vi "DCA Update Limit Listbox.vi"(6 "Colors":cluster{"Pass":u32, "Fail":u32, "Nop":u32}={"Pass"=6618880, "Fail"=16711680, "Nop"=16777226}, 7 "State (Pass/Fail)":enum16{"Reset", "In Progress", "Pass/Fail"}(ring)=enum."Pass/Fail", 8 "error in (no error)":errorcluster, 9 "Pass/Fail":bool[](array[boolean]), 10 "Limits":T1[](array[typedef]), 11 "Limit Status Ref":refnum<vi>) -> (0 "error out":errorcluster, 3 "Limit Status Ref Out":refnum<vi>)   [LabVIEW 2011]
uses:
  TypeDefs/DCA Limit.ctl
  TypeDefs/DCA Limit Quantity.ctl
  TypeDefs/DCA Limit Comparison.ctl
  TypeDefs/DCA Limit Operation.ctl
  Test Referential Limit.ctl
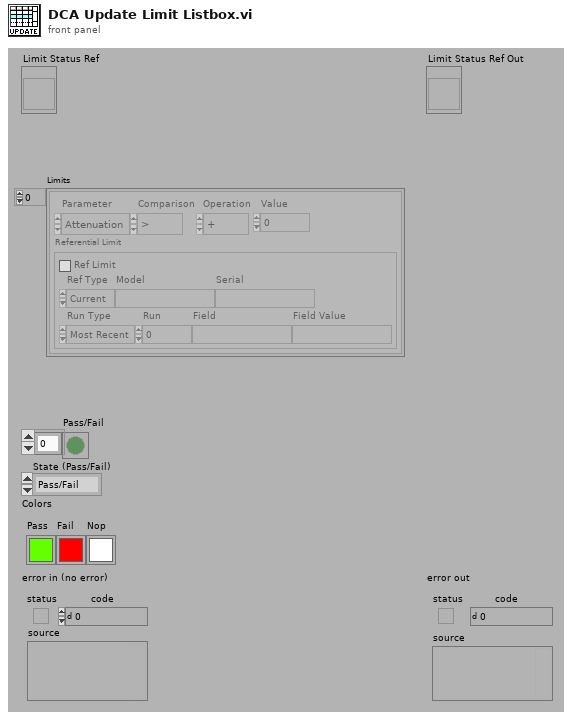
[diagram p1: front panel]
types:
  T1 = typedef "DCA Limit.ctl" = cluster{"Parameter":T2, "Comparison":T3, "Operation":T4, "Value":dbl, "Referential Limit":T5}
  T2 = typedef "DCA Limit Quantity.ctl" = enum16{"Attenuation", "Zin", "Zout", "R1", "R2", "R3", "Rab", "Rac", "Rbc"}
  T3 = typedef "DCA Limit Comparison.ctl" = enum16{">", ">=", "<", "<="}
  T4 = typedef "DCA Limit Operation.ctl" = enum16{"+", "-"}
  T5 = typedef "Test Referential Limit.ctl" = cluster{"Ref Limit":bool, "Ref Type":enum16{"Current", "Specify"}, "Model":string, "Serial":string, "Run Type":enum16{"Most Recent", "Run #", "Match Field"}, "Run":i32, "Field":string, "Field Value":string}
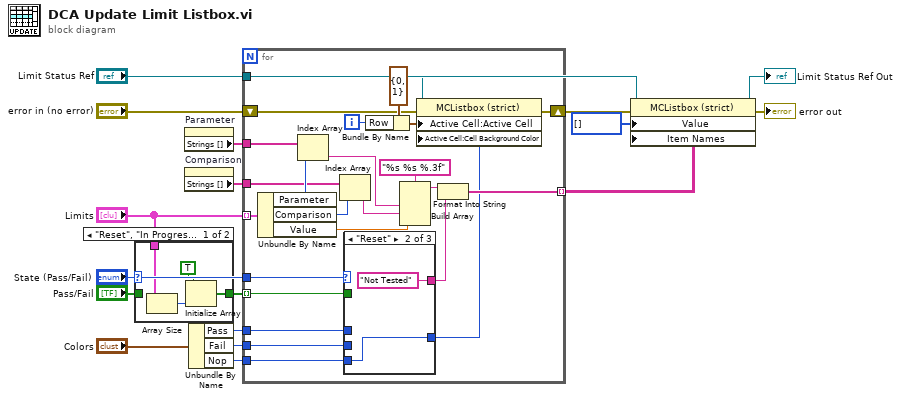
[diagram p0: block diagram]
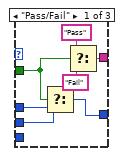
[diagram p3: hidden frame]
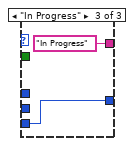
[diagram p4: hidden frame]
diagram:
  n1 = case shown="\"Reset\", \"In Progress\"" "State (Pass/Fail)" {
    tunnel: [w19 w22] -> w4
    tunnel: "Pass/Fail" -> [_ w22]
    tunnel: "Limits" -> [w18 _]
    frame "Reset", "In Progress" {
      n2 = Array Size(array=w18) -> (size(s)=w21:i32)
      n3 = Initialize Array(TRUE, w21) -> (w19:bool[])
    }
    frame "Pass/Fail" {
    }
  }
  n4 = property on="Parameter" class="Enum (strict)"() -> ("Strings []"=w9:string[])  [unwired: 2 in, 2 out]
  n5 = property on="Comparison" class="Enum (strict)"() -> ("Strings []"=w10:string[])  [unwired: 2 in, 2 out]
  n6 = Unbundle By Name("Colors") -> ("Pass"=w16:u32, "Fail"=w15:u32, "Nop"=w8:u32)
  n7 = for {
    tunnel: w16 -> [w27]
    tunnel: w15 -> [w26]
    tunnel: "Limit Status Ref" -> [w44]
    shift-right: [w42] -> w13
    shift-left: "error in (no error)" -> [w43]
    tunnel: "Limits" -> [w41] mode=indexing
    tunnel: [w39] -> w7 mode=indexing
    tunnel: w10 -> [w34]
    tunnel: w9 -> [w33]
    tunnel: w4 -> [w25] mode=indexing
    tunnel: w8 -> [w23]
    tunnel: "State (Pass/Fail)" -> [w24]
    i -> [w40]
    n8 = Unbundle By Name(w41) -> ("Parameter"=w35:T2, "Comparison"=w36:T3, "Value"=w30:dbl)
    n9 = Index Array(array=w33, index=w35) -> (element=w31:string)
    n10 = Index Array(array=w34, index=w36) -> (element=w32:string)
    n11 = case shown="\"Reset\"" w24 {
      tunnel: [w49 "Not Tested" "In Progress"] -> w29
      tunnel: [w53 w54 w56] -> w28
      tunnel: w27 -> [w52 _ _]
      tunnel: w26 -> [w51 _ _]
      tunnel: w25 -> [w50 _ _]
      tunnel: w23 -> [_ w54 w56]
      frame "Pass/Fail" {
        n12 = Select(t=w52, s=w50, f=w51) -> (s? t:f=w53:u32)
        n13 = Select(t="Pass" ("format string"), s=w50, f="Fail" ("format string")) -> (s? t:f=w49:string)
      }
      frame "Reset" {
      }
      frame "In Progress" {
      }
    }
    n14 = Bundle By Name(cluster=cluster{"Row":i32, "Column":i32} {"Row"=0, "Column"=1} ("Active Cell"), "Row"=w40) -> (w45:cluster{"Row":i32, "Column":i32})
    n15 = Format Into String(format string="%s %s %.3f", w31, w32, w30) -> (resulting string=w37:string)  [unwired: 2 in, 1 out]
    n16 = property class="MCListbox (strict)"(reference=w44, error in=w43, "Active Cell:Active Cell"=w45, "Active Cell:Cell Background Color"=w28) -> (error out=w42:errorcluster)  [unwired: 1 out]
    n17 = Build Array(w37, w29) -> (w39:string[])
  }
  n18 = property class="MCListbox (strict)"(reference="Limit Status Ref", error in=w13, "Value"=i32[] [], "Item Names"=w7) -> (reference out=→"Limit Status Ref Out":refnum<vi>, error out=→"error out":errorcluster)
